vi "Agilent N6900 N7900 Series Output Volt Arbitrary Waveform.vi"() -> ()   [LabVIEW 2021]
doc: "This example demonstrates configuring and running a voltage-based arbitrary waveform."
uses:
  <instrlib>/Agilent N6900 N7900 Series/Public/Configure/Arbitrary Waveform/Configure Arbitrary Waveform (Voltage).vi
  <instrlib>/Agilent N6900 N7900 Series/Agilent N6900 N7900 Series.lvlib
panel:
  in  "Voltage Points  (Blank)":dbl[](array[numeric])=[1.0, 2.0, 3.0, 4.0, 3.0, 2.0, 1.0]
  in  "stop":bool
  in  "Dwell Time (0.001)":dbl=0.001
  in  "VISA resource name":refnum<visa-resource-name>
  # "(c) 2013-2018 National Instruments Corporation.  ALL RIGHTS RESERVED."
  # "Outputs an arbitrary\nwaveform by providing an\narray of arbitrary amplitudes \nand the dwell time at each.\n\nBy default, this will output a\ntriangle wave."
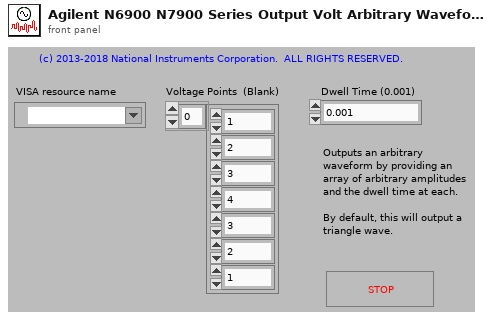
[diagram p1: front panel]
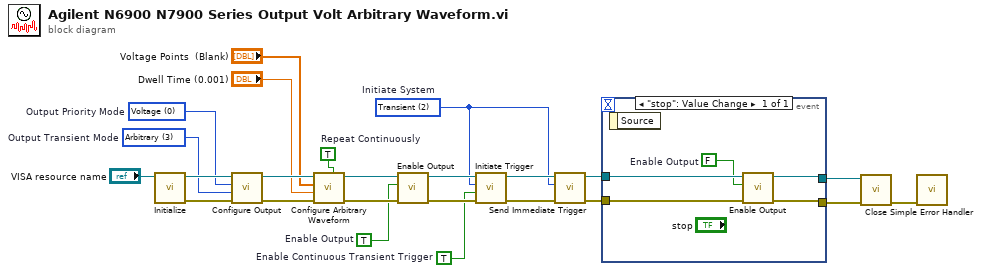
[diagram p0: block diagram]
diagram:
  w1 = TRUE  # Enable Output
  w7 = TRUE  # Repeat Continuously
  w10 = TRUE  # Enable Continuous Transient Trigger
  w9 = u16 2 items=["Acquisition", "External Logging", "Transient"]  # Initiate System
  w20 = u16 3 items=["Fixed", "Step", "List", "Arbitrary"]  # Output Transient Mode
  w21 = u16 0 items=["Voltage", "Current"]  # Output Priority Mode
  n1 = call <instrlib>:"Initialize.vi"("VISA resource name"="VISA resource name") -> ("error out"=w22:errorcluster, "VISA resource name out"=w23:refnum<visa-resource-name>)  [unwired: 9 in]
  n2 = call <instrlib>:"Configure Output.vi"("error in (no error)"=w22, "Output Transient Mode (0: Fixed)"=w20, "Output Priority Mode (0: Voltage)"=w21, "VISA resource name"=w23) -> ("error out"=w18:errorcluster, "VISA resource name out"=w19:refnum<visa-resource-name>)  [unwired: 6 in]
  n3 = call-poly <instrlib>:"Configure Arbitrary Waveform.vi"("Repeat Continuously (False)"=w7, "error in (no error)"=w18, "Dwell Time (0.001)"="Dwell Time (0.001)", "Voltage Points  (Blank)"="Voltage Points  (Blank)", "VISA resource name"=w19) -> ("error out"=w15:errorcluster, "VISA resource name out"=w16:refnum<visa-resource-name>)  [unwired: 5 in]
  n4 = call <instrlib>:"Enable Output.vi"("error in (no error)"=w15, "Enable Output (F: Disable)"=w1, "VISA resource name"=w16) -> ("error out"=w13:errorcluster, "VISA resource name out"=w14:refnum<visa-resource-name>)  [unwired: 7 in]
  n5 = call <instrlib>:"Initiate Trigger.vi"("error in (no error)"=w13, "Enable Continuous Transient Trigger (T: Enable)"=w10, "Initiate System (0: Acquisition)"=w9, "VISA resource name"=w14) -> ("error out"=w12:errorcluster, "VISA resource name out"=w11:refnum<visa-resource-name>)  [unwired: 6 in]
  n6 = call <instrlib>:"Send Immediate Trigger.vi"("error in (no error)"=w12, "Trigger System (0: Acquisition)"=w9, "VISA resource name"=w11) -> ("error out"=w5:errorcluster, "VISA resource name out"=w6:refnum<visa-resource-name>)  [unwired: 7 in]
  n7 = event shown="[0] \"stop\": Value Change" {
    selector: _ -> [_]
    dyn-events: _ -> [_]
    timeout: _ -> [_]
    tunnel: w6 -> [w29]
    tunnel: w5 -> [w26]
    tunnel: [w28] -> w4
    tunnel: [w27] -> w3
    event "stop": Value Change {
      w25 = FALSE  # Enable Output
      n8 = event-data() -> ()  [unwired: 1 in, 1 out]
      n9 = call <instrlib>:"Enable Output.vi"("error in (no error)"=w26, "Enable Output (F: Disable)"=w25, "VISA resource name"=w29) -> ("error out"=w27:errorcluster, "VISA resource name out"=w28:refnum<visa-resource-name>)  [unwired: 7 in]
    }
  }
  n10 = call <instrlib>:"Close.vi"("error in (no error)"=w3, "VISA resource name"=w4) -> ("error out"=w8:errorcluster)  [unwired: 9 in]
  n11 = call <vilib>:"Simple Error Handler.vi"("error in (no error)"=w8) -> ()  [unwired: 4 in, 5 out]
